vi "SetCtrlPropGenSgl.vi"(4 "Error in":errorcluster, 6 "Énum":T1(ring), 7 "Controls":refnum<vi>) -> (0 "Error out":errorcluster, 3 "Controls Out":refnum<vi>)   [LabVIEW 2012]
doc: "Ce VI ouvre le fichier de sauvegarde des modèles et lit les positions du modèle spécifié."
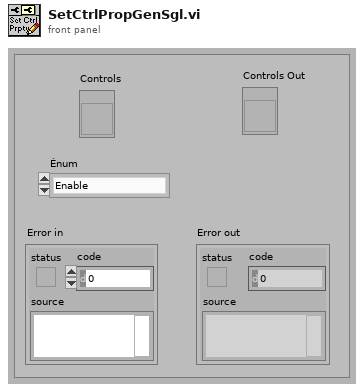
[diagram p1: front panel]
types:
  T1 = enum16{"Enable", "Disable", "DisAndGrayed", "ReinitToDefVal", "EnumElementsArr"}
  T2 = enum8{"Enabled", "Disabled", "Disabled and Grayed Out"}
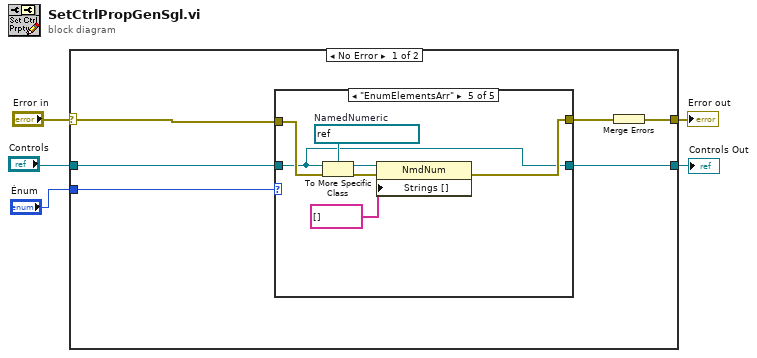
[diagram p0: block diagram]
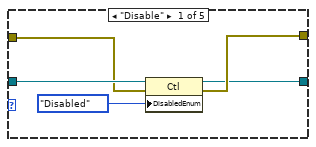
[diagram p2: hidden frame]
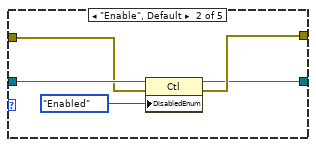
[diagram p3: hidden frame]
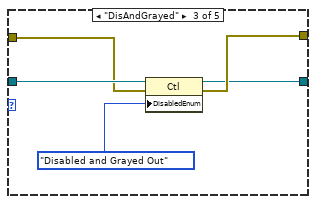
[diagram p4: hidden frame]
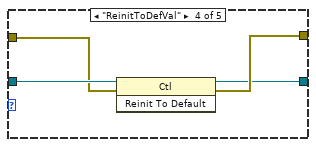
[diagram p5: hidden frame]
diagram:
  n1 = case shown="No Error" "Error in" {
    selector: "Error in" -> [w11 w38]
    tunnel: [w9 w38] -> w5
    tunnel: [w8 w37] -> w3
    tunnel: "Controls" -> [w7 w37]
    tunnel: "Énum" -> [w6 _]
    frame No Error {
      n2 = case shown="\"EnumElementsArr\"" w6 {
        tunnel: w7 -> [w16 w21 w26 w30 w31]
        tunnel: w11 -> [w14 w19 w24 w29 w36]
        tunnel: [w13 w18 w23 w28 w35] -> w10
        tunnel: [w12 w17 w22 w27 w31] -> w8
        frame "Disable" {
          n3 = property class="Ctl"(reference=w16, error in=w14, "DisabledEnum"=T2."Disabled" ("Désactivé")) -> (reference out=w12:refnum<vi>, error out=w13:errorcluster)
        }
        frame "Enable", Default {
          n4 = property class="Ctl"(reference=w21, error in=w19, "DisabledEnum"=T2."Enabled" ("Désactivé")) -> (reference out=w17:refnum<vi>, error out=w18:errorcluster)
        }
        frame "DisAndGrayed" {
          n5 = property class="Ctl"(reference=w26, error in=w24, "DisabledEnum"=T2."Disabled and Grayed Out" ("Désactivé")) -> (reference out=w22:refnum<vi>, error out=w23:errorcluster)
        }
        frame "ReinitToDefVal" {
          n6 = invoke class="Ctl" method="Reinit To Default"(reference=w30, error in=w29) -> (reference out=w27:refnum<vi>, error out=w28:errorcluster)  [unwired: 1 in, 1 out]
        }
        frame "EnumElementsArr" {
          w33 = refnum<vi> refnum  # NamedNumeric
          n7 = To More Specific Class(target class=w33, reference=w31) -> (specific class reference=w34:refnum<vi>)  [unwired: 1 in, 1 out]
          n8 = property class="NmdNum"(reference=w34, error in=w36, "Strings []"=string[] [] ("Noms d'éléments")) -> (error out=w35:errorcluster)  [unwired: 1 out]
        }
      }
      n9 = Merge Errors(w10) -> (w9:errorcluster)
    }
    frame Error {
    }
  }
  "Error out" <- w5
  "Controls Out" <- w3
